vi "Create Pattern Script(Addr_4W).vi"(8 "error in (no error)":errorcluster, 11 "Addr":u16 format="%x") -> (0 "error out":errorcluster, 3 "String":string)   [LabVIEW 2018, in "SPI_Frame_Root.lvclass"]
uses:
  SPI_Frame_Root.lvclass
  Classes/BML_Frame_Root/BML_Frame_Root.lvclass
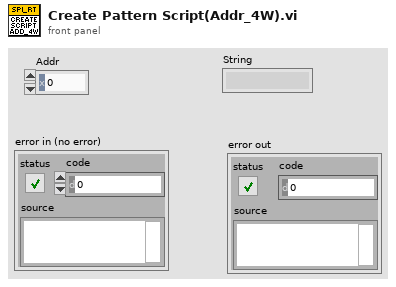
[diagram p1: front panel]
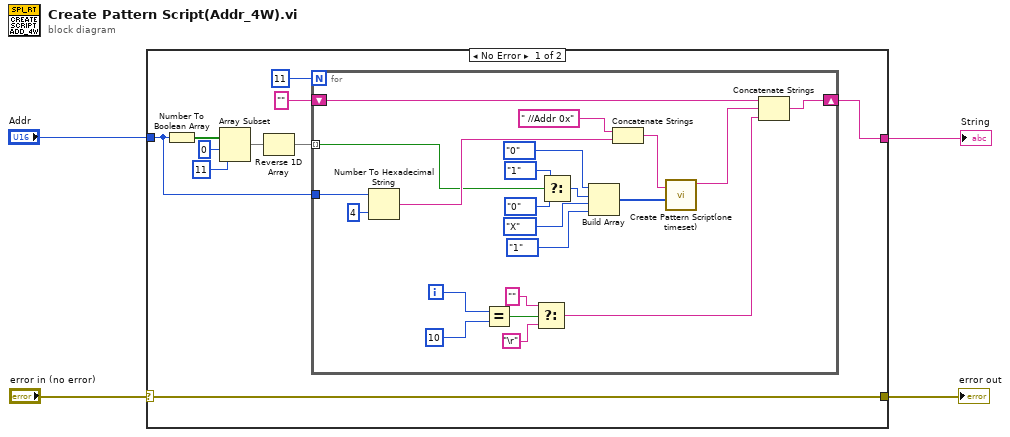
[diagram p0: block diagram]
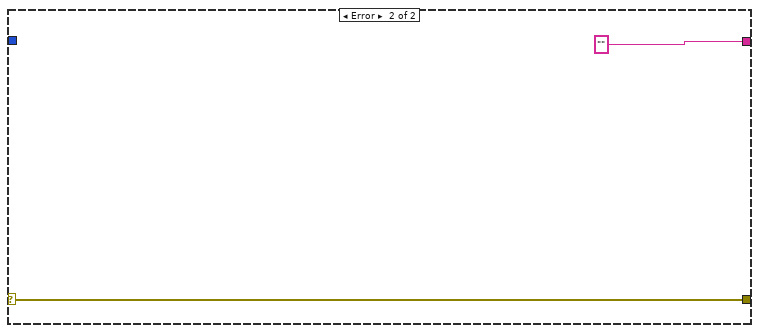
[diagram p2: hidden frame]
diagram:
  n1 = case shown="No Error" "error in (no error)" {
    selector: "error in (no error)" -> [w14 w37]
    tunnel: [w11 ""] -> w3
    tunnel: [w14 w37] -> w2
    tunnel: "Addr" -> [w10 _]
    frame No Error {
      n2 = Number To Boolean Array(number=w10) -> (Boolean array=w9:bool[])
      n3 = Array Subset(array=w9, index=0, length=11) -> (w6:bool[])
      n4 = Reverse 1D Array(array=w6) -> (reversed array=w5:bool[])
      n5 = for {
        N: 11 -> [_]
        shift-right: [w31] -> w11
        shift-left: "" -> [w30]
        tunnel: w10 -> [w29]
        tunnel: w5 -> [w20] mode=indexing
        i -> [w21]
        n6 = Number To Hexadecimal String(1:i16 4 ("width (-)"), 2:w29) -> (0:w27:string)
        n7 = Equal?(x=w21, y=10) -> (x = y?=w35:bool)
        n8 = Select(t="", s=w35, f="\r") -> (s? t:f=w32:string)
        n9 = Select(t=enum16{"0", "1", "L", "H", "X", "V", "D", "M"}."1" ("PinState"), s=w20, f=enum16{"0", "1", "L", "H", "X", "V", "D", "M"}."0") -> (s? t:f=w17:enum16{"0", "1", "L", "H", "X", "V", "D", "M"})
        n10 = Build Array(enum16{"0", "1", "L", "H", "X", "V", "D", "M"}."0" ("element"), w17, enum16{"0", "1", "L", "H", "X", "V", "D", "M"}."X" ("element"), enum16{"0", "1", "L", "H", "X", "V", "D", "M"}."1" ("element")) -> (w25:enum16{"0", "1", "L", "H", "X", "V", "D", "M"}[])
        n11 = Concatenate Strings(" //Addr 0x" ("Notes"), w27) -> (w22:string)
        n12 = call "Create Pattern Script(one timeset).vi"("Notes"=w22, "PinState"=w25) -> ("string out"=w19:string)  [unwired: 9 in]
        n13 = Concatenate Strings(w30, w19, w32) -> (w31:string)
      }
    }
    frame Error {
    }
  }
  "String" <- w3
  "error out" <- w2
